vi "case_struct_add_sub.vi"() -> ()   [LabVIEW 2026]
panel:
  in  "ON/OFF":bool
  out "OUTPUT":dbl
  in  "NUM 2":dbl
  in  "NUM 1":dbl
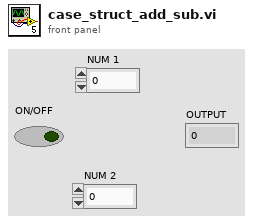
[diagram p1: front panel]
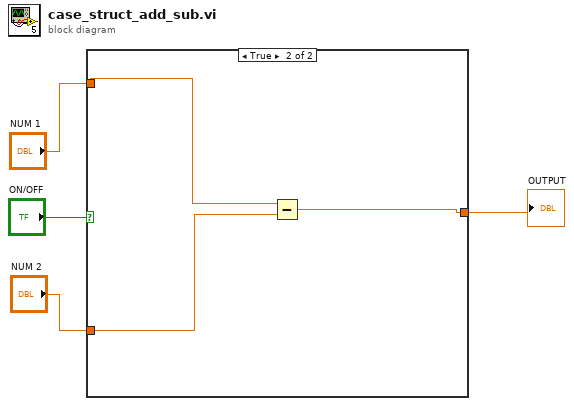
[diagram p0: block diagram]
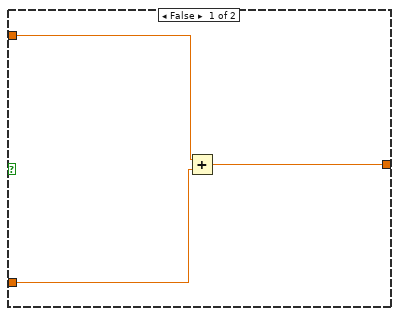
[diagram p2: hidden frame]
diagram:
  n1 = case shown="True" "ON/OFF" {
    tunnel: "NUM 1" -> [w7 w10]
    tunnel: "NUM 2" -> [w6 w9]
    tunnel: [w5 w8] -> w1
    frame False {
      n2 = Add(x=w7, y=w6) -> (x+y=w5:dbl)
    }
    frame True {
      n3 = Subtract(x=w10, y=w9) -> (x-y=w8:dbl)
    }
  }
  "OUTPUT" <- w1
